vi "Read stl file, build and save octree.vi"(0 "STL file path (load)":path, 1 "String":string, 2 "Model rotation axis (unit vector)":sgl[](array[numeric]), 5 "Auto resolution":bool=TRUE, 7 "Specify resolution":sgl=100.0, 9 "Invert model (interior region)":bool, 11 "Model Rotation (deg)":sgl, 12 "Model rotation axis coordinates (absolute, mm)":sgl[](array[numeric])) -> (3 "Octree node array":T2[](array[typedef]), 4 "Octree resolution":sgl, 13 "Error out":errorcluster, 14 "Triangles array":T1[](array[typedef]))   [LabVIEW 2018]
uses:
  Typedefs/TreeNodeBox.ctl
  Typedefs/Quad.ctl
  Typedefs/Quadplane enum.ctl
  Typedefs/Triangle.ctl
panel:
  # "PN 23/01/2015"
  # "Vertices"
  # "Edges"
  # "Unit normal"
  # "Edge unit normals"
  # "Vertices"
  # "Edges"
  # "Unit normal"
  # "Plane ident."
  # "Vertices"
  # "Edges"
  # "Unit normal"
  # "Plane ident."
  # "Vertices"
  # "Edges"
  # "Unit normal"
  # "Plane ident."
  # "Vertices"
  # "Edges"
  # "Unit normal"
  # "Plane ident."
  # "Vertices"
  # "Edges"
  # "Unit normal"
  # "Plane ident."
  # "Vertices"
  # "Edges"
  # "Unit normal"
  # "Plane ident."
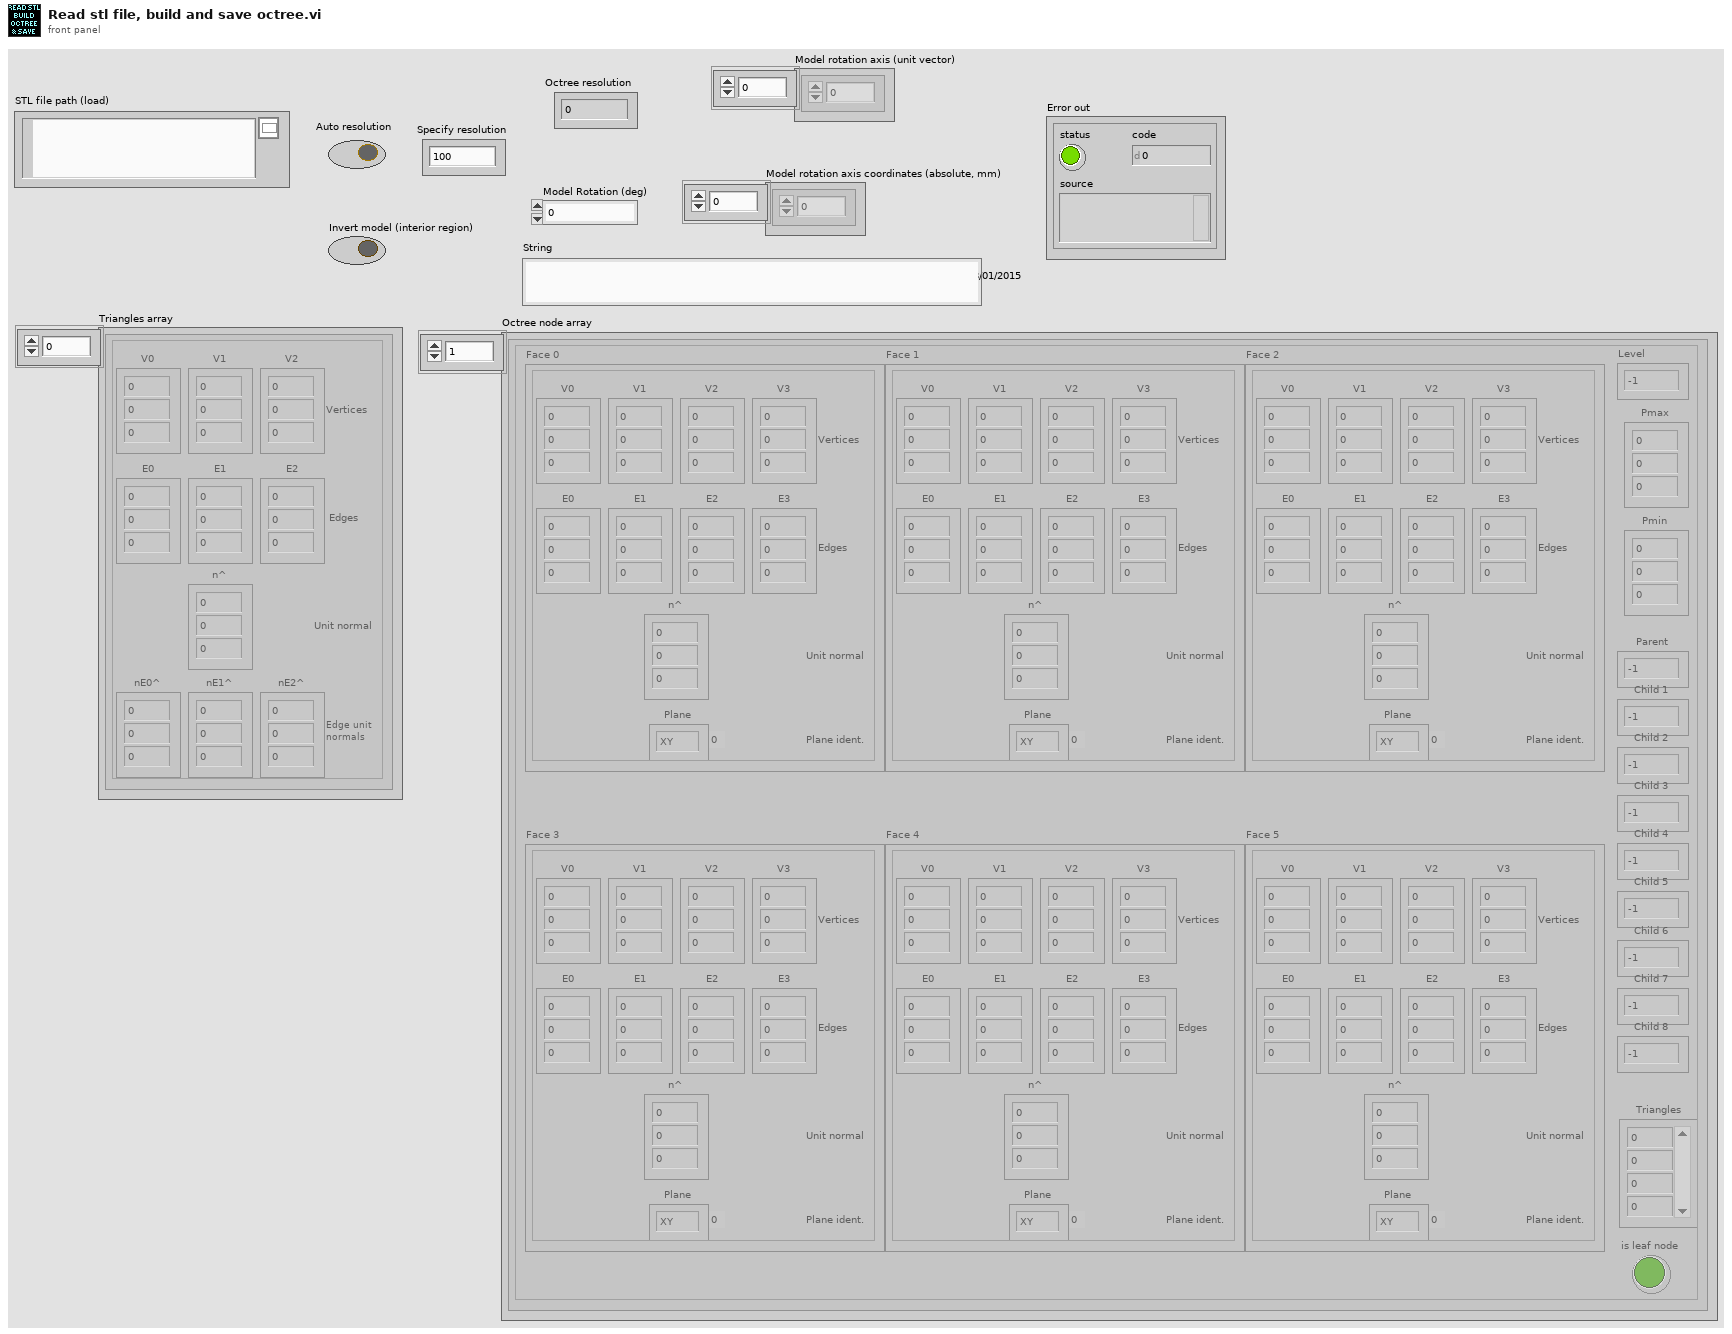
[diagram p1: front panel]
types:
  T1 = typedef "Triangle.ctl" = cluster{"V0":sgl[], "V1":sgl[], "V2":sgl[], "E0":sgl[], "E1":sgl[], "E2":sgl[], "n^":sgl[], "nE0^":sgl[], "nE1^":sgl[], "nE2^":sgl[]}
  T2 = typedef "TreeNodeBox.ctl" = cluster{"Face 0":T3, "Face 1":T3, "Face 2":T3, "Face 3":T3, "Face 4":T3, "Face 5":T3, "Level":i32, "Pmax":sgl[], "Pmin":sgl[], "Parent":i32, "Child 1":i32, "Child 2":i32, "Child 3":i32, "Child 4":i32, "Child 5":i32, "Child 6":i32, "Child 7":i32, "Child 8":i32, "Triangles":i32[], "is leaf node":bool}
  T3 = typedef "Quad.ctl" = cluster{"V0":sgl[], "V1":sgl[], "V2":sgl[], "V3":sgl[], "E0":sgl[], "E1":sgl[], "E2":sgl[], "E3":sgl[], "n^":sgl[], "Plane":T4}
  T4 = typedef "Quadplane enum.ctl" = enum8{"XY", "XZ", "YZ", "-XY", "-XZ", "-YZ"}
  T5 = cluster{"Specify resolution":sgl, "Invert model (interior region)":bool, "STL file path (load)":path, "Model rotation axis (unit vector)":sgl[], "Model rotation axis coordinates (absolute, mm)":sgl[], "Model Rotation (deg)":sgl}
  T6 = cluster{"Specify resolution":sgl, "Invert model (interior region)":bool, "STL file path (load)":path, "Model rotation axis (unit vector)":sgl[], "Model rotation axis coordinates (absolute, mm)":sgl[], "Model Rotation (deg)":sgl}[]
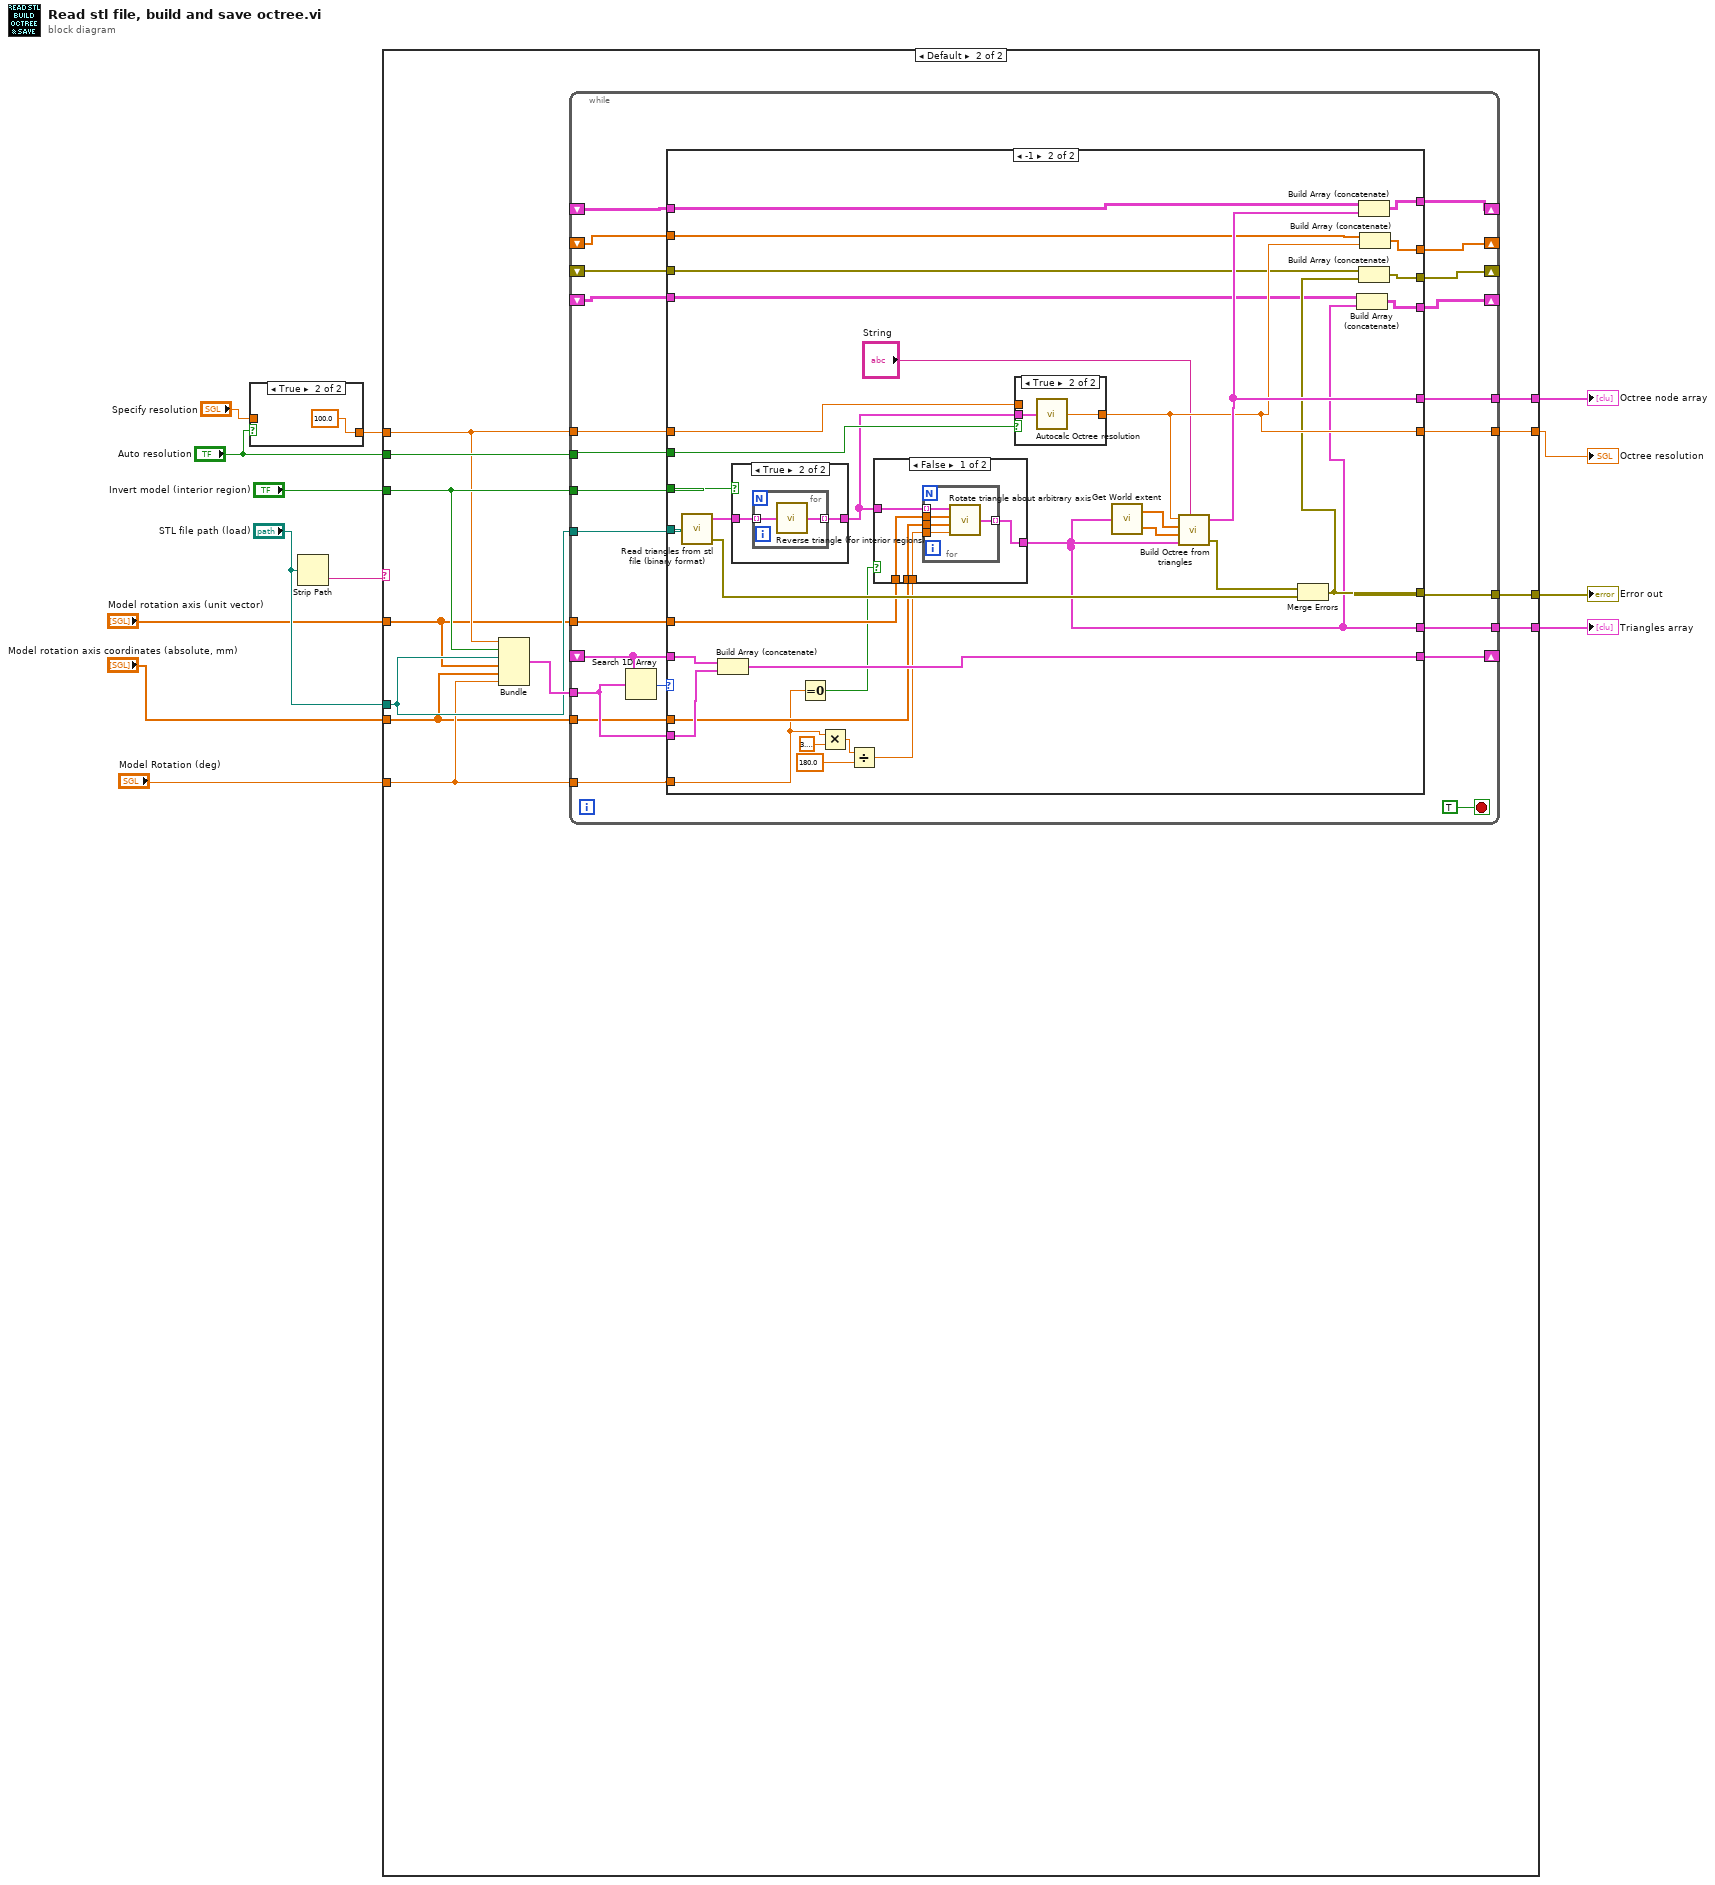
[diagram p0: block diagram]
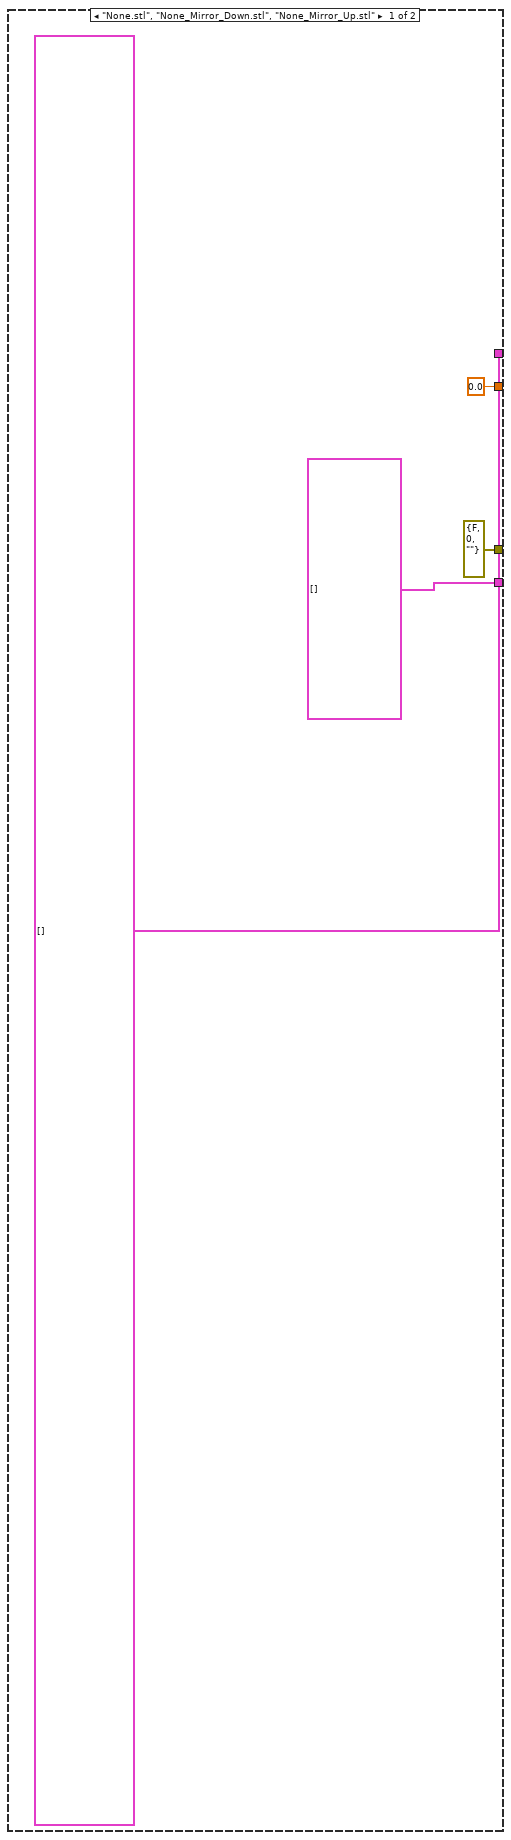
[diagram p3: hidden frame]
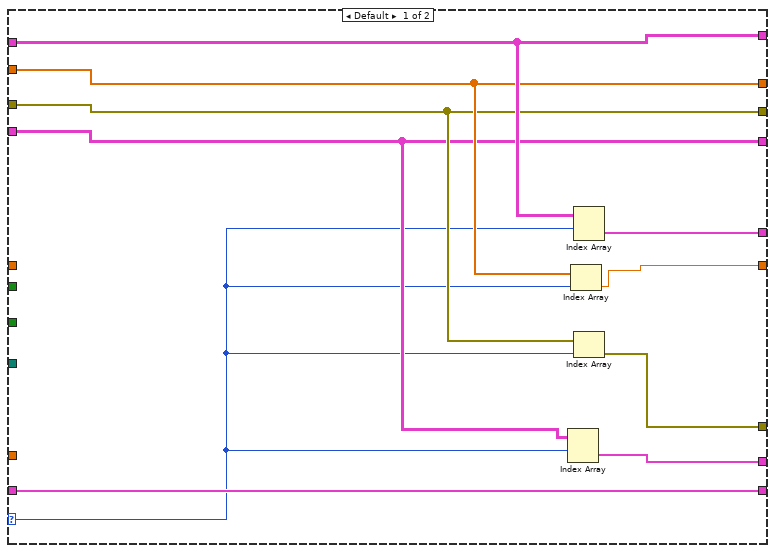
[diagram p4: hidden frame]
diagram:
  n1 = case shown="True" "Auto resolution" {
    tunnel: "Specify resolution" -> [w14 _]
    tunnel: [w14 sgl 100.0 ("Specify resolution")] -> w1
    frame False {
    }
    frame True {
    }
  }
  n2 = Strip Path(path="STL file path (load)") -> (name=w7:string)  [unwired: 1 out]
  n3 = case shown="Default" w7 {
    tunnel: [T2[] [] ("Octree node array") w31] -> w13
    tunnel: [errorcluster {"status"=FALSE, "code"=0, "source"=""} ("error IO") w30] -> w12
    tunnel: [T1[] [] ("Triangles array") w29] -> w11
    tunnel: "Auto resolution" -> [_ w28]
    tunnel: "Invert model (interior region)" -> [_ w27]
    tunnel: w1 -> [_ w26]
    tunnel: [sgl 0.0 ("Suggested resolution") w25] -> w9
    tunnel: "STL file path (load)" -> [_ w23]
    tunnel: "Model rotation axis (unit vector)" -> [_ w20]
    tunnel: "Model rotation axis coordinates (absolute, mm)" -> [_ w21]
    tunnel: "Model Rotation (deg)" -> [_ w22]
    frame "None.stl", "None_Mirror_Down.stl", "None_Mirror_Up.stl" {
    }
    frame Default {
      n4 = Bundle("Specify resolution"=w26, "Invert model (interior region)"=w27, "STL file path (load)"=w23, "Model rotation axis (unit vector)"=w20, "Model rotation axis coordinates (absolute, mm)"=w21, "Model Rotation (deg)"=w22) -> (w24:T5)  [unwired: 1 in]
      n5 = while {
        tunnel: [w55] -> w31
        tunnel: [w54] -> w30
        tunnel: [w53] -> w29
        tunnel: w28 -> [w52]
        tunnel: w27 -> [w51]
        tunnel: w23 -> [w50]
        tunnel: w26 -> [w49]
        tunnel: [w48] -> w25
        shift-right: [w40] -> _
        shift-left: _ -> [w41]
        shift-right: [w44] -> _
        shift-left: _ -> [w46]
        tunnel: w24 -> [w45]
        shift-right: [w42] -> _
        shift-left: _ -> [w43]
        shift-right: [w39] -> _
        shift-left: _ -> [w37]
        shift-right: [w38] -> _
        shift-left: _ -> [w36]
        tunnel: w20 -> [w34]
        tunnel: w21 -> [w33]
        tunnel: w22 -> [w32]
        stop <- TRUE stop-if-true
        n6 = Search 1D Array(1D array=w46, element=w45) -> (index of element=w47:i32)  [unwired: 1 in]
        n7 = case shown="-1" w47 {
          selector: w47 -> [w58 _]
          tunnel: [w63 w87] -> w55
          tunnel: [w56 w79] -> w54
          tunnel: [w57 w68] -> w53
          tunnel: w52 -> [_ w94]
          tunnel: w51 -> [_ w93]
          tunnel: w50 -> [_ w92]
          tunnel: w49 -> [_ w91]
          tunnel: [w61 w80] -> w48
          tunnel: w46 -> [w65 w90]
          tunnel: w45 -> [_ w89]
          tunnel: [w65 w88] -> w44
          tunnel: w43 -> [w64 w86]
          tunnel: [w64 w85] -> w42
          tunnel: w41 -> [w62 w84]
          tunnel: [w62 w83] -> w40
          tunnel: [w60 w82] -> w39
          tunnel: [w59 w81] -> w38
          tunnel: w37 -> [w60 w78]
          tunnel: w36 -> [w59 w77]
          tunnel: w34 -> [_ w74]
          tunnel: w33 -> [_ w73]
          tunnel: w32 -> [_ w67]
          frame Default {
            n8 = Index Array(array=w59, index (row)=w58) -> (element=w57:T1[])  [unwired: 1 in]
            n9 = Index Array(array=w62, index=w58) -> (element=w61:sgl)
            n10 = Index Array(array=w64, index (row)=w58) -> (element=w63:T2[])  [unwired: 1 in]
            n11 = Index Array(array=w60, index=w58) -> (element=w56:errorcluster)
          }
          frame -1 {
            n12 = call "Read triangles from stl file (binary format).vi"("STL file path"=w92) -> ("Triangles array"=w97:T1[], "Error out"=w96:errorcluster)  [unwired: 1 out]
            n13 = Build Array (concatenate)(w90, w89) -> (w88:T6)
            n14 = case shown="True" w93 {
              tunnel: w97 -> [w111 w113]
              tunnel: [w111 w112] -> w75
              frame False {
              }
              frame True {
                n15 = for {
                  tunnel: w113 -> [w115] mode=indexing
                  tunnel: [w114] -> w112 mode=indexing
                  n16 = call "Reverse triangle (for interior regions).vi"("Triangle in"=w115) -> ("Triangle out"=w114:T1)
                }
              }
            }
            n17 = Equal To 0?(x=w67) -> (x = 0?=w66:bool)
            n18 = Multiply(x=w67, y=sgl 3.1415927) -> (x*y=w72:sgl)
            n19 = Divide(x=w72, y=sgl 180.0) -> (x/y=w69:sgl)
            n20 = case shown="False" w66 {
              tunnel: w75 -> [w104 w110]
              tunnel: w74 -> [w103 _]
              tunnel: w73 -> [w102 _]
              tunnel: w69 -> [w101 _]
              tunnel: [w100 w110] -> w68
              frame False {
                n21 = for {
                  tunnel: w104 -> [w109] mode=indexing
                  tunnel: w103 -> [w108]
                  tunnel: w101 -> [w107]
                  tunnel: [w105] -> w100 mode=indexing
                  tunnel: w102 -> [w106]
                  n22 = call "Rotate triangle about arbitrary axis.vi"("Rotation angle (rad)"=w107, "Rotation axis coordinates (x, y, z)"=w106, "Rotation axis (unit direction vector)\nanti-clockwise positive looking into axis"=w108, "Triangle in"=w109) -> ("Triangle out"=w105:T1)
                }
              }
              frame True {
              }
            }
            n23 = case shown="True" w94 {
              tunnel: [w116 w118] -> w80
              tunnel: w75 -> [_ w117]
              tunnel: w91 -> [w116 _]
              frame False {
              }
              frame True {
                n24 = call "Autocalc Octree resolution.vi"("Triangles array"=w117) -> ("Suggested resolution"=w118:sgl)
              }
            }
            n25 = call "Get World extent.vi"("Triangles"=w68) -> ("Pmax (x, y, z)"=w99:sgl[], "Pmin (x, y, z)"=w98:sgl[])
            n26 = call "Build Octree from triangles.vi"("Octree resolution (model units)"=w80, "World Pmax (x, y, z)"=w99, "World Pmin (x, y, z)"=w98, "Triangle array"=w68, "String"="String") -> ("Octree node array"=w87:T2[], "Stack error"=w95:errorcluster)  [unwired: 1 out]
            n27 = Merge Errors(w95, w96) -> (w79:errorcluster)
            n28 = Build Array (concatenate)(w77, w68) -> (w81:T1[][])
            n29 = Build Array (concatenate)(w86, w87) -> (w85:T2[][])
            n30 = Build Array (concatenate)(w78, w79) -> (w82:errorcluster[])
            n31 = Build Array (concatenate)(w84, w80) -> (w83:sgl[])
          }
        }
      }
    }
  }
  "Octree resolution" <- w9
  "Error out" <- w12
  "Octree node array" <- w13
  "Triangles array" <- w11
